vi "Clockwise.Reverse Global.vi"() -> ()   [LabVIEW 2014, in "Main Libraryv2.lvlib"]
uses:
  Control/Main Libraryv2.lvlib
panel:
  in  "Clockwise/Reverse":bool
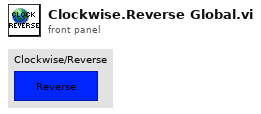
[diagram p1: front panel]
diagram:
